vi "Section and key name.vi"() -> ()   [LabVIEW 2017]
panel:
  in  "Row4 Match ROI":string="Row4 Match ROI"
  in  "Row3 Match ROI":string="Row3 Match ROI"
  in  "Row2 Match ROI":string="Row2 Match ROI"
  in  "Find Center ROI":string="Find Center ROI"
  in  "Row1 Match ROI":string="Row1 Match ROI"
  in  "Find Ering ROI":string="Find Ering ROI"
  # "section item name"
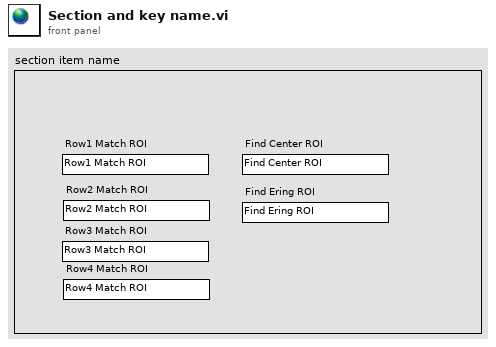
[diagram p1: front panel]
diagram:
